vi "DCS(Dual_Inst).vi"(3 "error in":errorcluster) -> (10 "error out":errorcluster)   [LabVIEW 2013]
uses:
  <vilib>/Utility/miscctls.llb/LVPointTypeDef.ctl
  <userlib>/Accelerator/User Interface/Controls/Role ID.ctl
panel:
  out "Changed front panel":bool
  in  "stop":bool
  in  "Tab Control":enum32{"Engineering Graphs", "Maintenance"}(tab)
  out "DCS 2 Second Plane":ext[][](graph)
  out "DCS 2 First Plane":ext[][](graph)
  out "DCS 1 Second Plane":ext[][](graph)
  out "DCS 1 First Plane":ext[][](graph)
  out "DCS 1 Signals":ext[][](graph)
  out "DCS 2 Signals":ext[][](graph)
  out "Aquisition Rate Value 2":i64
  out "Aquisition Rate Value 1":i64
  out "DAQ 1 Sample Size Window":u32
  in  "DAQ 1 Trim Time":dbl=0.0001
  in  "DAQ 2 Trim Time":dbl=0.0001
  out "DAQ 2 Sample Size Window":i32
  in  "Save Waveforms":bool
  in  "Posttrigger size 2":i32=50000
  in  "Acquisition Rate 2":u16(ring)=2 items=["40 MHz", "20 MHz", "10 MHz", "5 MHz", "2.5 MHz", "1 MHz", "100 kHz", "10 kHz"]
  in  "Pretrigger size 2":i32=1
  in  "Rising or falling? 2":bool
  in  "Jorger 2 TR slot":i32=6
  out "Sampling Frequency":u16(ring) items=["40 MHz", "20 MHz", "10 MHz", "5 MHz", "2.5 MHz", "1 MHz", "100 kHz", "10 kHz"]
  out "Length of Sample":dbl caption="s" format="%^#_3g"
  out "Memory Address Pointer":ext
  out "Post trigger Size":ext
  out "Pretrigger Size":ext
  out "Trigger Generation register":i32=23 format="%.0b"
  out "status register":i8=4 format="%08b"
  out "control register":i16=23 format="%015b"
  in  "Posttrigger size":i32=1
  in  "Acquisition Rate":u16(ring)=2 items=["40 MHz", "20 MHz", "10 MHz", "5 MHz", "2.5 MHz", "1 MHz", "100 kHz", "10 kHz"]
  in  "Pretrigger size":i32=60000
  in  "Rising or falling?":bool
  out "Running Errors":errorcluster
  in  "Jorger 1 TR slot":i32=3
  in  "Joerger 1 Channels":i32[](array[numeric])=[0, 1, 2, 3, 4, 5, 6, 9]
  in  "Joerger 2 Channels":i32[](array[numeric])=[0, 1, 2, 3, 4, 6, 7, 8]
  out "control register 2":i16=23 format="%015b"
  out "status register 2":i8=4 format="%08b"
  out "Memory Address Pointer 2":ext
  out "Post trigger Size 2":ext
  out "Pretrigger Size 2":ext
  out "Sampling Frequency 2":u16(ring) items=["40 MHz", "20 MHz", "10 MHz", "5 MHz", "2.5 MHz", "1 MHz", "100 kHz", "10 kHz"]
  # "Ensure Joeger Card Channels are functional.\nDefault values should reflect this."
  # "Rising or falling? not functional. Ignore"
  # "DAQ 2 Parameter Controls"
  # "Falling"
  # "Rising"
  # "DAQ Parameter Indicators"
  # "DAQ 1 Parameter Controls"
  # "Falling"
  # "Rising"
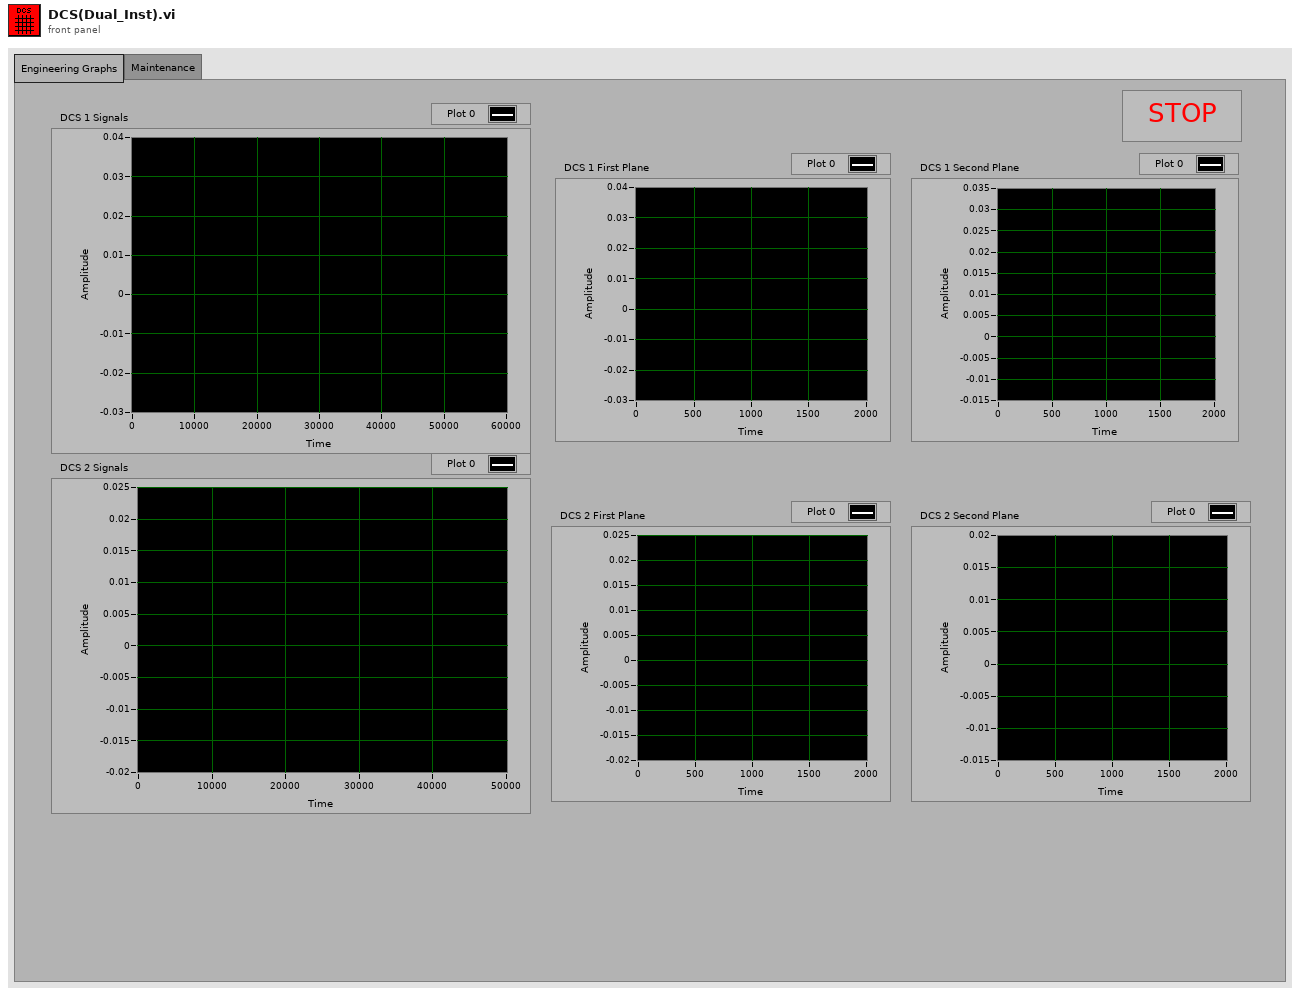
[diagram p1: front panel]
types:
  T1 = typedef "LVPointTypeDef.ctl" = cluster{"Horizontal":i16, "Vertical":i16}
  T2 = typedef "Role ID.ctl" = enum16{"First_Detector", "Second_Detector", "Third_Detector", "LeCroy_CH1", "LeCroy_CH2", "LeCroy_CH3", "LeCroy_CH4", "PSU", "DCS 1", "DCS 2"}
  T3 = enum32{"DCS", "Spot Size Tracking", "Engineering Graphs", "Maintenance"}
  T4 = cluster{"Data":dbl[][], "Integer Timestamp":u64, "Signal Length":u32, "DCS ID":u64, "Role ID":T2}
  T5 = cluster{"Data":dbl[][], "Integer Timestamp":u64, "Signal Length":u32, "DCS ID":u64, "Role ID":T2}[]
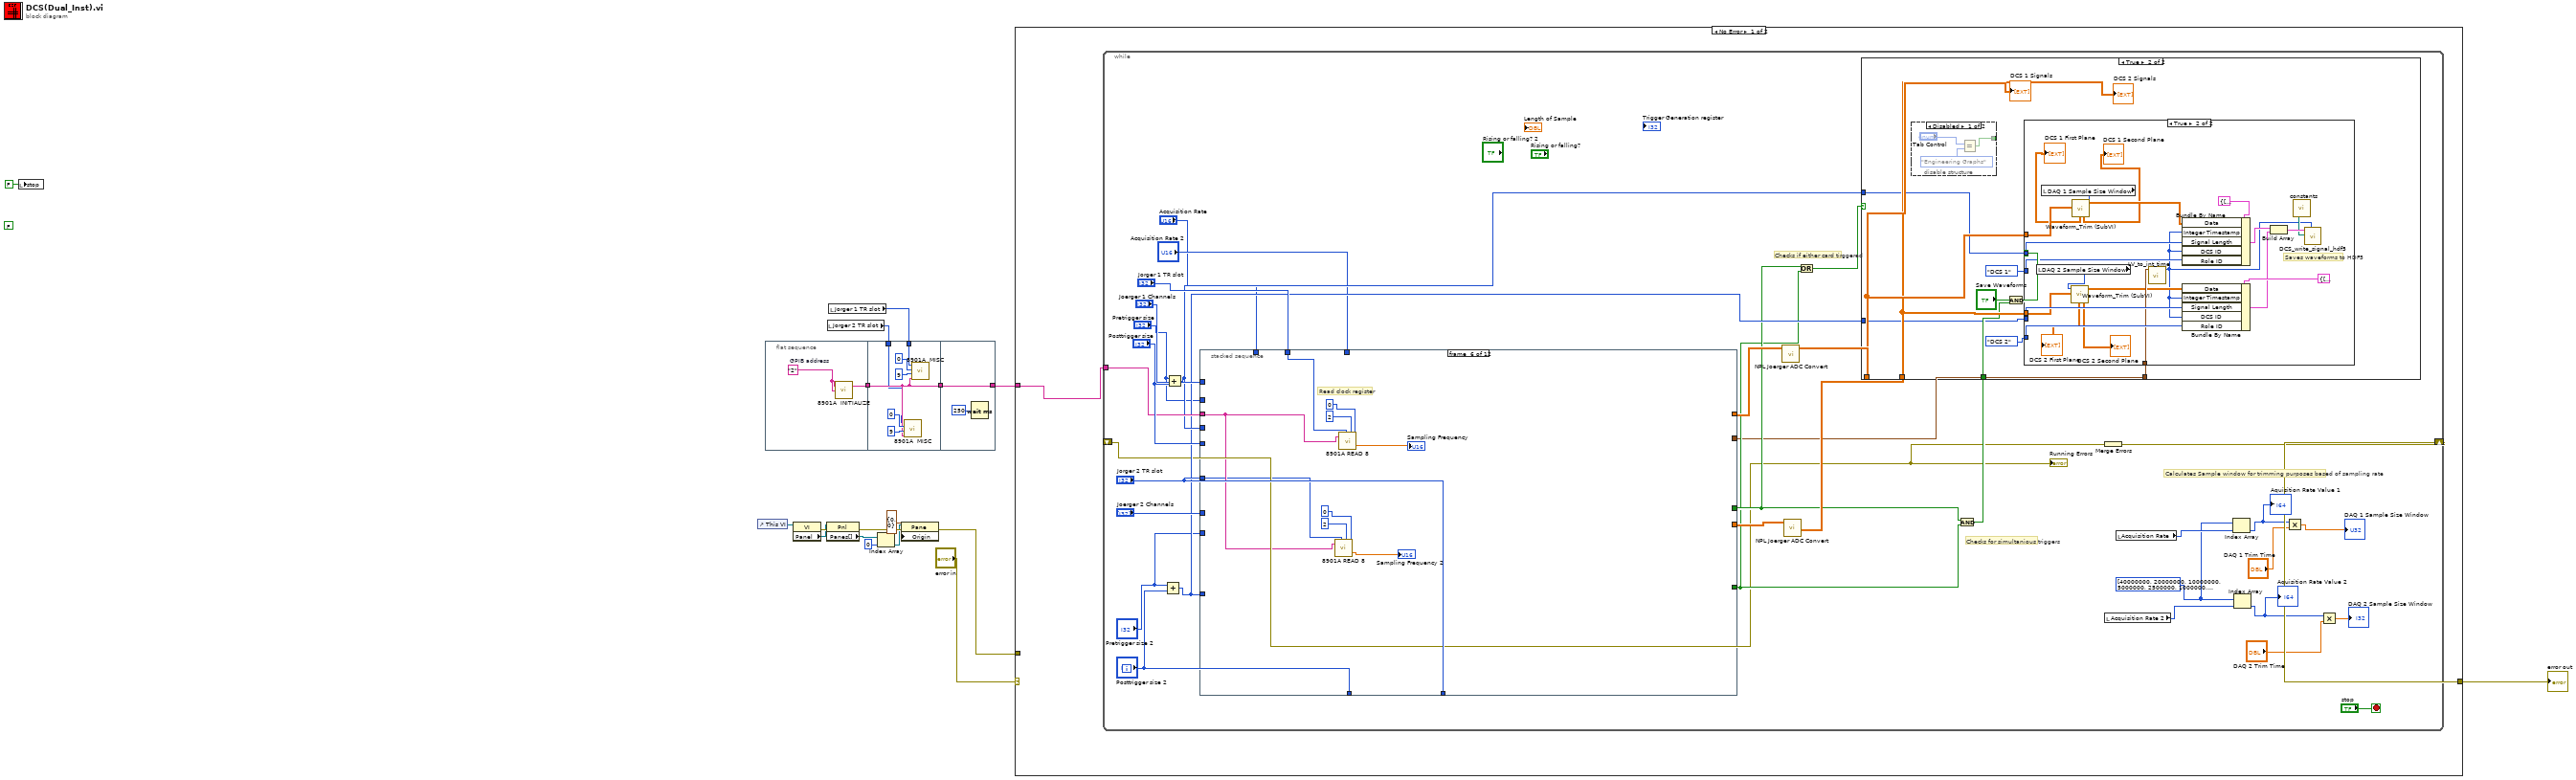
[diagram p0: block diagram]
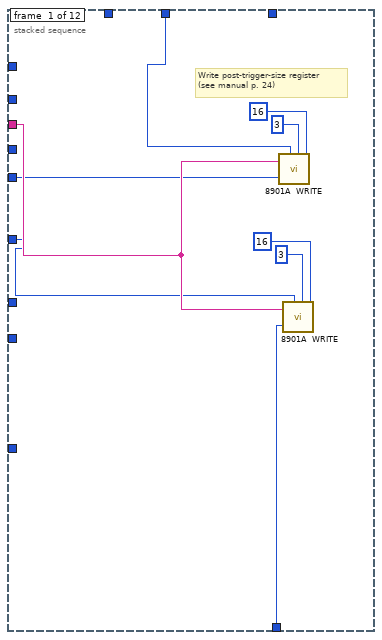
[diagram p5: hidden frame]
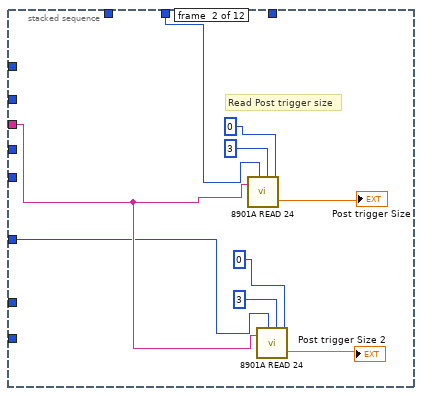
[diagram p6: hidden frame]
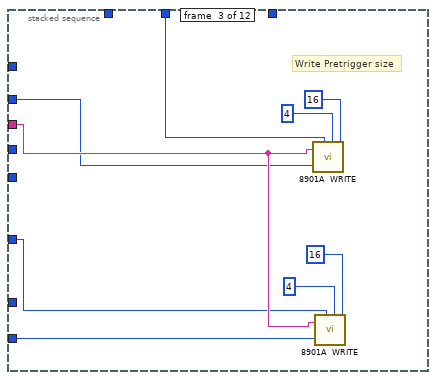
[diagram p7: hidden frame]
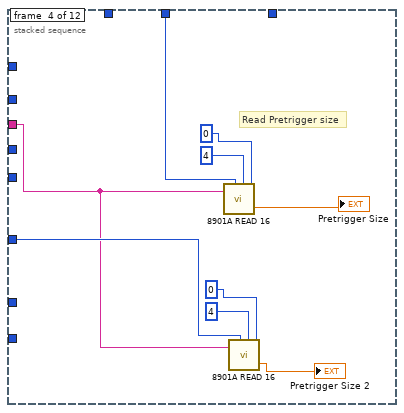
[diagram p8: hidden frame]
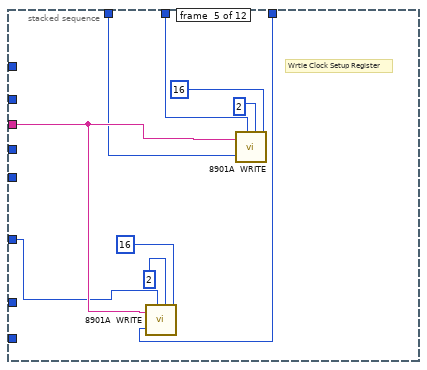
[diagram p9: hidden frame]
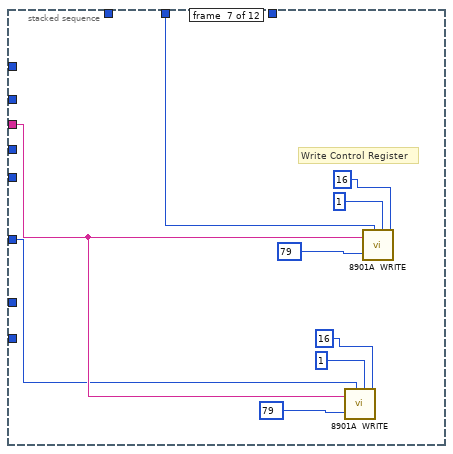
[diagram p10: hidden frame]
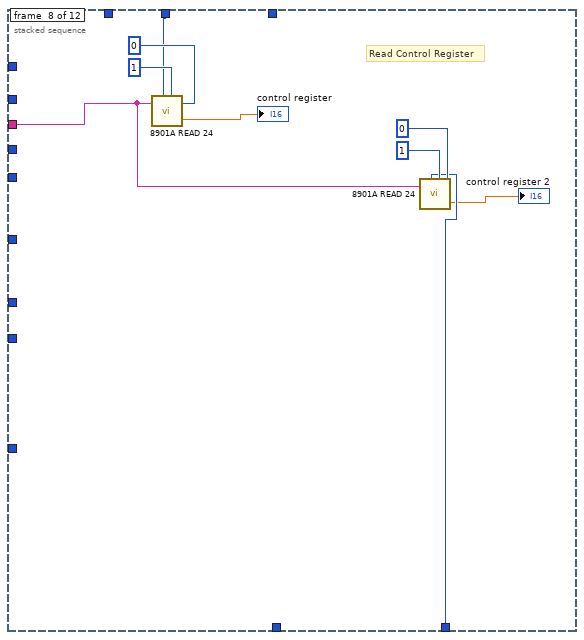
[diagram p11: hidden frame]
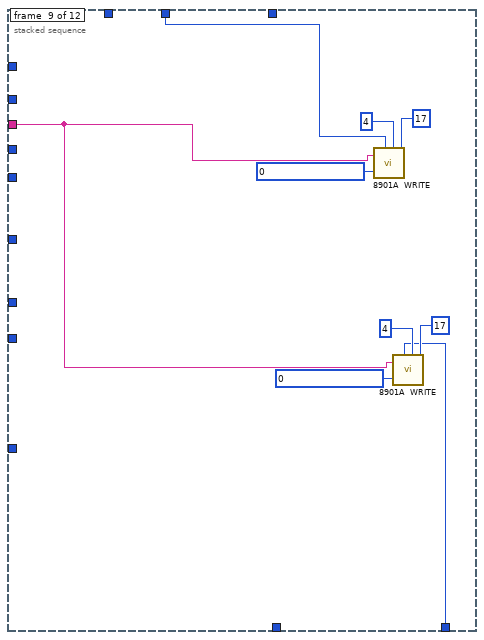
[diagram p12: hidden frame]
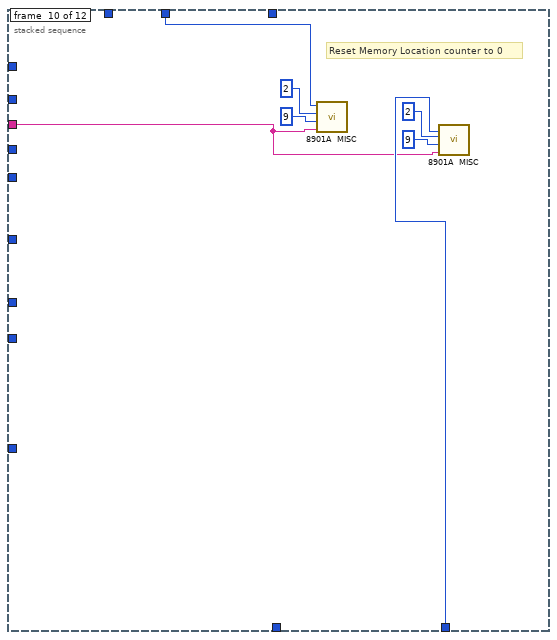
[diagram p13: hidden frame]
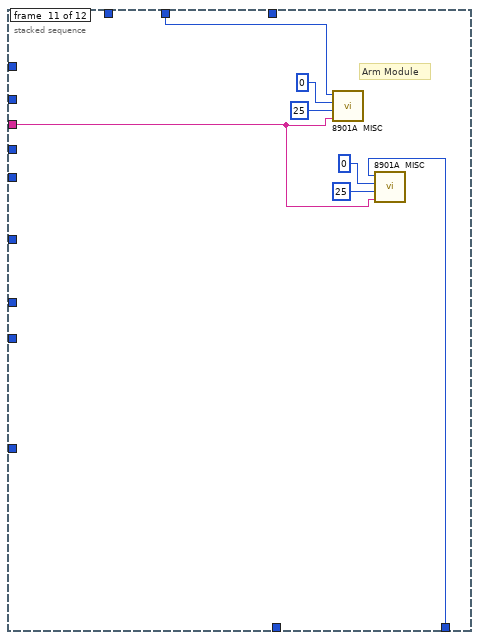
[diagram p14: hidden frame]
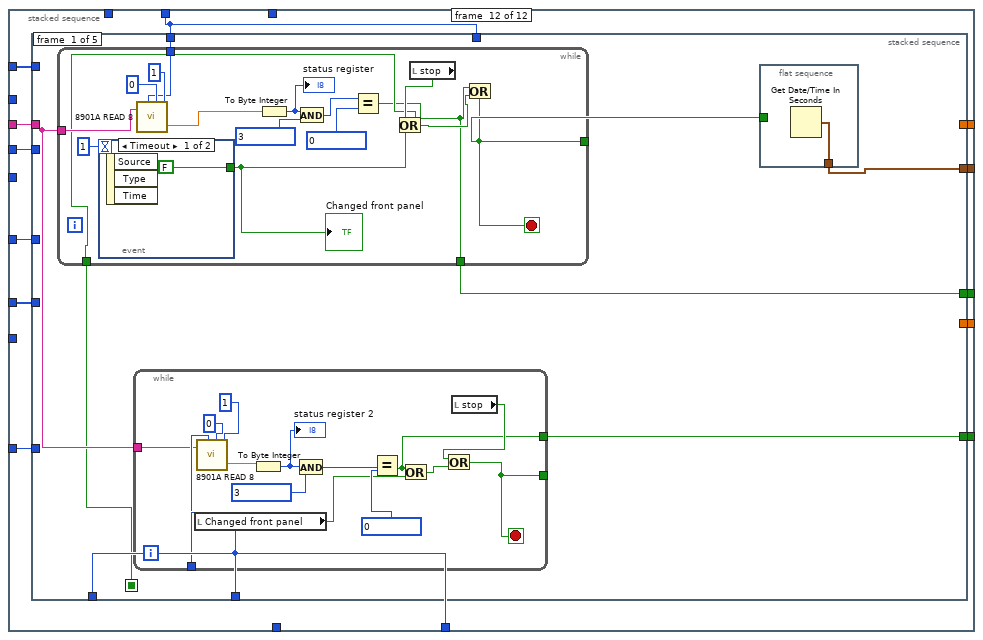
[diagram p15: hidden frame]
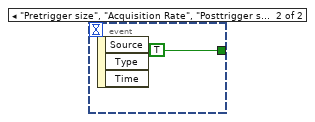
[diagram p16: hidden frame]
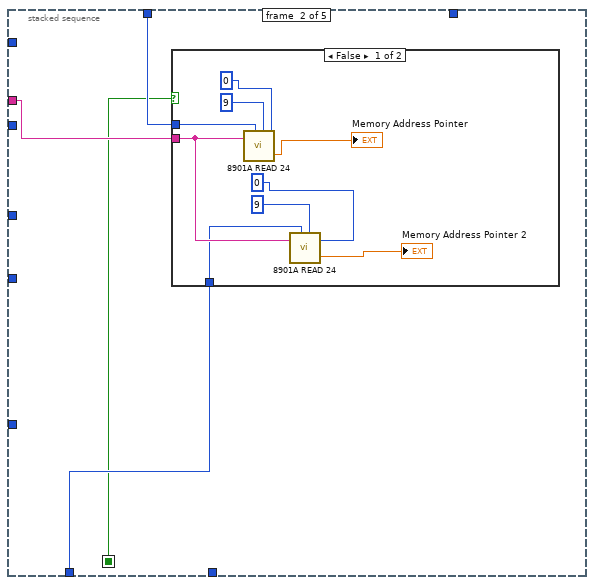
[diagram p17: hidden frame]
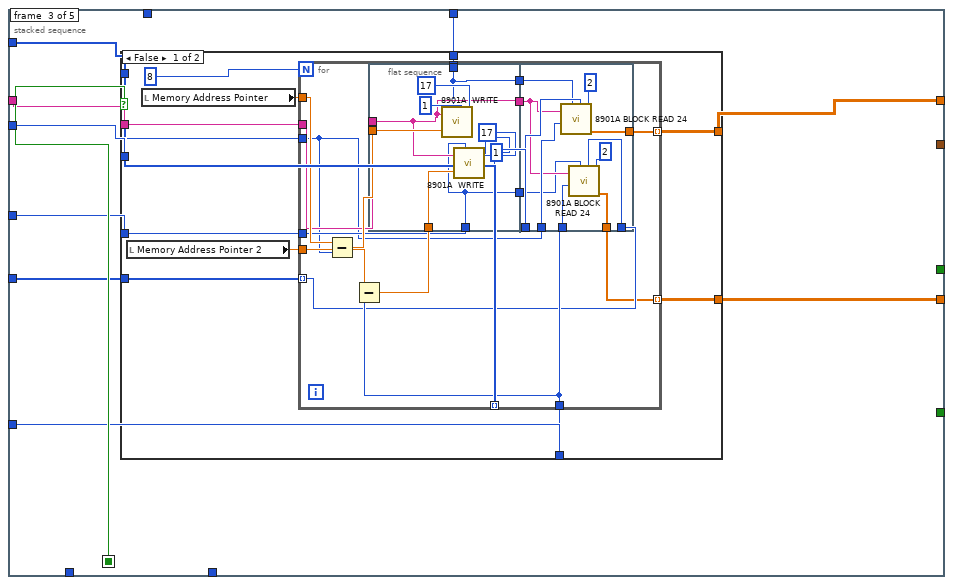
[diagram p19: hidden frame]
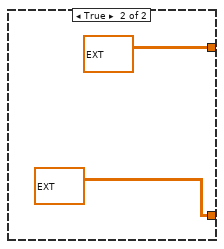
[diagram p20: hidden frame]
diagram:
  (unwired) FALSE ("Auto Threshold")
  n1 = local write "stop"(FALSE ("stop")) -> ()
  n2 = control-ref of="This VI"() -> (w14:refnum<vi>)
  n3 = flat-sequence {
    tunnel: [w18] -> w4
    tunnel: w4 -> [w21]
    tunnel: w3 -> [w20]
    tunnel: w2 -> [w19]
    tunnel: [w21] -> w1
    tunnel: [w27] -> w5
    tunnel: w1 -> [w27]
    frame #0 {
      w18 = "2"  # GPIB address
      n4 = call <instrlib>:"8901A  INITIALIZE.vi"("GPIB address"=w18) -> ()
    }
    frame #1 {
      n5 = call <instrlib>:"8901A  MISC.vi"("GPIB address"=w21, "f"=9, "a"=0, "n"=w19) -> ()
      n6 = call <instrlib>:"8901A  MISC.vi"("GPIB address"=w21, "f"=9, "a"=0, "n"=w20) -> ()
    }
    frame #2 {
      n7 = Wait (ms)(milliseconds to wait=250) -> ()  [unwired: 1 out]
    }
  }
  n8 = property class="VI"(reference=w14) -> (error out=w13:errorcluster, "Panel"=w12:refnum<vi>)  [unwired: 1 in, 1 out]
  n9 = property class="Pnl"(reference=w12, error in=w13) -> (error out=w11:errorcluster, "Panes[]"=w10:refnum<vi>[])  [unwired: 1 out]
  n10 = local read "Jorger 2 TR slot"() -> (w2:i32)
  n11 = local read "Jorger 1 TR slot"() -> (w3:i32)
  n12 = Index Array(array=w10, index=0) -> (element=w8:refnum<vi>)
  n13 = property class="Pane"(reference=w8, error in=w11, "Origin"=T1 {"Horizontal"=0, "Vertical"=0}) -> (error out=w6:errorcluster)  [unwired: 1 out]
  n14 = case shown="No Error" "error in" {
    selector: "error in" -> [_ w336]
    tunnel: [w29 w336] -> w16
    tunnel: w6 -> [_ _]
    tunnel: w5 -> [w28 _]
    frame No Error {
      n15 = while {
        shift-right: [w32] -> w29
        shift-left: _ -> [w33]
        tunnel: w28 -> [w53]
        stop <- "stop" stop-if-true
        w36 = i32[] [40000000, 20000000, 10000000, 5000000, 2500000, 1000000, 100000, 10000]
        # "Calculates Sample window for trimming purposes based of sampling rate"
        # "Checks if either card tirggered"
        # "Checks for simultanious triggers"
        n16 = Add(x="Pretrigger size 2", y="Posttrigger size 2") -> (x+y=w50:i32)
        n17 = Add(x="Pretrigger size", y="Posttrigger size") -> (x+y=w51:i32)
        n18 = stacked-sequence {
          tunnel: w53 -> [w103 w114 w121 w126 w139 w150 w154 w165 w173 w185 w189 w203]
          tunnel: w51 -> [_ _ _ _ _ _ _ _ _ _ _ w206]
          tunnel: "Joerger 1 Channels" -> [_ _ _ _ _ _ _ _ _ _ _ w205]
          tunnel: [_ _ _ _ _ _ _ _ _ _ _ w204] -> w61
          tunnel: "Jorger 2 TR slot" -> [_ _ _ _ _ _ _ w164 w171 w186 w188 w202]
          tunnel: "Jorger 1 TR slot" -> [w102 w110 w120 w130 w138 w148 w158 w162 w172 w184 w187 w195]
          tunnel: "Jorger 2 TR slot" -> [w101 w111 w119 w129 w137 w147 w153 _ _ _ _ w200]
          tunnel: "Posttrigger size" -> [w100 _ _ _ _ _ _ _ _ _ _ _]
          tunnel: "Posttrigger size 2" -> [w99 _ _ _ _ _ _ _ _ _ _ _]
          tunnel: "Acquisition Rate" -> [_ _ _ _ w136 _ _ _ _ _ _ _]
          tunnel: "Acquisition Rate 2" -> [_ _ _ _ w135 _ _ _ _ _ _ _]
          tunnel: w50 -> [_ _ _ _ _ _ _ _ _ _ _ w201]
          tunnel: "Joerger 2 Channels" -> [_ _ _ _ _ _ _ _ _ _ _ w199]
          tunnel: [_ _ _ _ _ _ _ _ _ _ _ w198] -> w52
          tunnel: [_ _ _ _ _ _ _ _ _ _ _ w197] -> w48
          tunnel: [_ _ _ _ _ _ _ _ _ _ _ w196] -> w47
          tunnel: "Pretrigger size 2" -> [_ _ w118 _ _ _ _ _ _ _ _ _]
          tunnel: "Pretrigger size" -> [_ _ w117 _ _ _ _ _ _ _ _ _]
          tunnel: [_ _ _ _ _ _ _ _ _ _ _ w194] -> w41
          frame #0 {
            # "Write post-trigger-size register\n(see manual p. 24)"
            n19 = call <instrlib>:"8901A  WRITE.vi"("data"=w100, "GPIB address"=w103, "n"=w102, "a"=3, "f"=16) -> ()  [unwired: 1 in]
            n20 = call <instrlib>:"8901A  WRITE.vi"("data"=w99, "GPIB address"=w103, "n"=w101, "a"=3, "f"=16) -> ()  [unwired: 1 in]
          }
          frame #1 {
            # "Read Post trigger size"
            n21 = call <instrlib>:"8901A READ 24.vi"("GPIB address"=w114, "n"=w110, "a"=3, "f"=0) -> ("output"=→"Post trigger Size":ext)  [unwired: 3 in]
            n22 = call <instrlib>:"8901A READ 24.vi"("GPIB address"=w114, "n"=w111, "a"=3, "f"=0) -> ("output"=→"Post trigger Size 2":ext)  [unwired: 3 in]
          }
          frame #2 {
            # "Write Pretrigger size"
            n23 = call <instrlib>:"8901A  WRITE.vi"("data"=w117, "GPIB address"=w121, "n"=w120, "a"=4, "f"=16) -> ()  [unwired: 1 in]
            n24 = call <instrlib>:"8901A  WRITE.vi"("data"=w118, "GPIB address"=w121, "n"=w119, "a"=4, "f"=16) -> ()  [unwired: 1 in]
          }
          frame #3 {
            # "Read Pretrigger size"
            n25 = call <instrlib>:"8901A READ 16.vi"("GPIB address"=w126, "n"=w130, "a"=u8 4, "f"=u8 0) -> ("output"=→"Pretrigger Size":ext)  [unwired: 3 in]
            n26 = call <instrlib>:"8901A READ 16.vi"("GPIB address"=w126, "n"=w129, "a"=u8 4, "f"=u8 0) -> ("output"=→"Pretrigger Size 2":ext)  [unwired: 3 in]
          }
          frame #4 {
            # "Wrtie Clock Setup Register"
            n27 = call <instrlib>:"8901A  WRITE.vi"("data"=w135, "GPIB address"=w139, "n"=w137, "a"=2, "f"=16) -> ()  [unwired: 1 in]
            n28 = call <instrlib>:"8901A  WRITE.vi"("data"=w136, "GPIB address"=w139, "n"=w138, "a"=2, "f"=16) -> ()  [unwired: 1 in]
          }
          frame #5 {
            # "Read clock register"
            n29 = call <instrlib>:"8901A READ 8.vi"("GPIB address"=w150, "n"=w147, "a"=2, "f"=0) -> ("output"=→"Sampling Frequency 2":ext)  [unwired: 3 in]
            n30 = call <instrlib>:"8901A READ 8.vi"("GPIB address"=w150, "n"=w148, "a"=2, "f"=0) -> ("output"=→"Sampling Frequency":ext)  [unwired: 3 in]
          }
          frame #6 {
            # "Write Control Register"
            n31 = call <instrlib>:"8901A  WRITE.vi"("data"=79, "GPIB address"=w154, "n"=w153, "a"=1, "f"=16) -> ()  [unwired: 1 in]
            n32 = call <instrlib>:"8901A  WRITE.vi"("data"=79, "GPIB address"=w154, "n"=w158, "a"=1, "f"=16) -> ()  [unwired: 1 in]
          }
          frame #7 {
            # "Read Control Register"
            n33 = call <instrlib>:"8901A READ 24.vi"("GPIB address"=w165, "n"=w162, "a"=1, "f"=0) -> ("output"=→"control register":ext)  [unwired: 3 in]
            n34 = call <instrlib>:"8901A READ 24.vi"("GPIB address"=w165, "n"=w164, "a"=1, "f"=0) -> ("output"=→"control register 2":ext)  [unwired: 3 in]
          }
          frame #8 {
            n35 = call <instrlib>:"8901A  WRITE.vi"("data"=0, "GPIB address"=w173, "n"=w172, "a"=u8 4, "f"=u8 17) -> ()  [unwired: 1 in]
            n36 = call <instrlib>:"8901A  WRITE.vi"("data"=0, "GPIB address"=w173, "n"=w171, "a"=u8 4, "f"=u8 17) -> ()  [unwired: 1 in]
          }
          frame #9 {
            # "Reset Memory Location counter to 0"
            n37 = call <instrlib>:"8901A  MISC.vi"("GPIB address"=w185, "f"=u8 9, "a"=u8 2, "n"=w184) -> ()
            n38 = call <instrlib>:"8901A  MISC.vi"("GPIB address"=w185, "f"=u8 9, "a"=u8 2, "n"=w186) -> ()
          }
          frame #10 {
            # "Arm Module"
            n39 = call <instrlib>:"8901A  MISC.vi"("GPIB address"=w189, "f"=25, "a"=0, "n"=w187) -> ()
            n40 = call <instrlib>:"8901A  MISC.vi"("GPIB address"=w189, "f"=25, "a"=0, "n"=w188) -> ()
          }
          frame #11 {
            n41 = stacked-sequence {
              seq-local: [w212 _ _ _ _] -> [_ w247 w269 _ _]
              tunnel: w206 -> [_ _ w268 _ _]
              tunnel: w205 -> [_ _ w267 _ _]
              tunnel: [_ _ w265 _ _] -> w204
              tunnel: w202 -> [w214 _ _ w321 _]
              tunnel: w203 -> [w213 w250 w266 w322 w331]
              tunnel: w202 -> [_ w249 _ _ _]
              tunnel: w201 -> [_ _ w264 _ _]
              tunnel: w195 -> [_ _ w263 _ w330]
              tunnel: w200 -> [_ _ w261 _ w329]
              tunnel: w199 -> [_ _ w262 _ _]
              tunnel: [_ _ w260 _ _] -> w198
              tunnel: [w211 _ _ _ _] -> w197
              tunnel: [w210 _ _ _ _] -> w196
              tunnel: w195 -> [w209 w248 _ w325 _]
              tunnel: [w207 _ _ _ _] -> w194
              frame #0 {
                n42 = while {
                  tunnel: w213 -> [w237]
                  tunnel: [w235] -> w208
                  tunnel: [w231] -> w212
                  tunnel: [w230] -> w211
                  tunnel: w209 -> [w229]
                  stop <- w235 stop-if-true
                  n43 = event shown="[0] Timeout" {
                    selector: _ -> [_ _]
                    dyn-events: _ -> [_ _]
                    timeout: 1 -> [_ _]
                    tunnel: [FALSE TRUE] -> w233
                    event Timeout {
                      n44 = event-data() -> ()  [unwired: 1 in, 3 out]
                    }
                    event "Pretrigger size", "Acquisition Rate", "Posttrigger size", "control register": Value Change {
                      n45 = event-data() -> ()  [unwired: 1 in, 3 out]
                    }
                  }
                  "Changed front panel" <- w233
                  n46 = call <instrlib>:"8901A READ 8.vi"("GPIB address"=w237, "n"=w229, "a"=0, "f"=1) -> ("output"=w240:ext)  [unwired: 3 in]
                  n47 = To Byte Integer(number=w240) -> (8bit integer=w236:i8)
                  "status register" <- w236
                  n48 = And(x=w236, y=i8 3) -> (x .and. y?=w241:i8)
                  n49 = Equal?(x=w241, y=i8 0) -> (x = y?=w230:bool)
                  n50 = local read "stop"() -> (w232:bool)
                  n51 = Or(x=w232, y=w233) -> (x .or. y?=w231:bool)
                  n52 = Or(x=w230, y=w231) -> (x .or. y?=w235:bool)
                }
                n53 = while {
                  tunnel: w214 -> [w226]
                  tunnel: w213 -> [w225]
                  tunnel: [w218] -> _
                  tunnel: [w215] -> w210
                  stop <- w218 stop-if-true
                  n54 = local read "Changed front panel"() -> (w216:bool)
                  n55 = call <instrlib>:"8901A READ 8.vi"("GPIB address"=w225, "n"=w226, "a"=0, "f"=1) -> ("output"=w224:ext)  [unwired: 3 in]
                  n56 = To Byte Integer(number=w224) -> (8bit integer=w220:i8)
                  "status register 2" <- w220
                  n57 = And(x=w220, y=i8 3) -> (x .and. y?=w222:i8)
                  n58 = Equal?(x=w222, y=i8 0) -> (x = y?=w215:bool)
                  n59 = Or(x=w215, y=w216) -> (x .or. y?=w217:bool)
                  n60 = local read "stop"() -> (w219:bool)
                  n61 = Or(x=w219, y=w217) -> (x .or. y?=w218:bool)
                }
                n62 = flat-sequence {
                  tunnel: w208 -> [_]
                  tunnel: [w246] -> w207
                  frame #0 {
                    n63 = Get Date/Time In Seconds() -> (seconds since 1Jan1904=w246:timestamp)
                  }
                }
              }
              frame #1 {
                n64 = case shown="False" w247 {
                  tunnel: w250 -> [w254 _]
                  tunnel: w249 -> [w253 _]
                  tunnel: w248 -> [w251 _]
                  frame False {
                    n65 = call <instrlib>:"8901A READ 24.vi"("GPIB address"=w254, "n"=w251, "a"=u8 9, "f"=u8 0) -> ("output"=→"Memory Address Pointer":ext)  [unwired: 3 in]
                    n66 = call <instrlib>:"8901A READ 24.vi"("GPIB address"=w254, "n"=w253, "a"=u8 9, "f"=u8 0) -> ("output"=→"Memory Address Pointer 2":ext)  [unwired: 3 in]
                  }
                  frame True {
                  }
                }
              }
              frame #2 {
                n67 = case shown="False" w269 {
                  tunnel: w268 -> [w279 _]
                  tunnel: w267 -> [w280 _]
                  tunnel: w266 -> [w278 _]
                  tunnel: [w276 ext[][] [[nan]] ("output")] -> w265
                  tunnel: w264 -> [w275 _]
                  tunnel: w263 -> [w273 _]
                  tunnel: w261 -> [w272 _]
                  tunnel: w262 -> [w271 _]
                  tunnel: [w270 ext[][] [[nan]] ("output")] -> w260
                  frame False {
                    n68 = local read "Memory Address Pointer 2"() -> (w274:ext)
                    n69 = local read "Memory Address Pointer"() -> (w277:ext)
                    n70 = for {
                      N: 8 -> [_]
                      tunnel: w280 -> [w293] mode=indexing
                      tunnel: w279 -> [w284]
                      tunnel: w278 -> [w295]
                      tunnel: w277 -> [w297]
                      tunnel: [w292] -> w276 mode=indexing
                      tunnel: w275 -> [w290]
                      tunnel: w274 -> [w291]
                      tunnel: w273 -> [w288]
                      tunnel: w272 -> [w287]
                      tunnel: w271 -> [w283] mode=indexing
                      tunnel: [w282] -> w270 mode=indexing
                      n71 = Subtract(x=w297, y=w284) -> (x-y=w296:ext)
                      n72 = Subtract(x=w291, y=w290) -> (x-y=w289:ext)
                      n73 = flat-sequence {
                        tunnel: w296 -> [w304]
                        tunnel: w295 -> [w302]
                        tunnel: [w302] -> w294
                        tunnel: w289 -> [w303]
                        tunnel: w288 -> [w298]
                        tunnel: w287 -> [w299]
                        tunnel: [w298] -> w286
                        tunnel: [w299] -> w285
                        tunnel: w294 -> [w310]
                        tunnel: w293 -> [w312]
                        tunnel: w284 -> [w316]
                        tunnel: [w315] -> w292
                        tunnel: w290 -> [w313]
                        tunnel: w286 -> [w307]
                        tunnel: w285 -> [w308]
                        tunnel: w283 -> [w311]
                        tunnel: [w309] -> w282
                        frame #0 {
                          n74 = call <instrlib>:"8901A  WRITE.vi"("data"=w304, "GPIB address"=w302, "n"=w298, "a"=1, "f"=17) -> ()  [unwired: 1 in]
                          n75 = call <instrlib>:"8901A  WRITE.vi"("data"=w303, "GPIB address"=w302, "n"=w299, "a"=1, "f"=17) -> ()  [unwired: 1 in]
                        }
                        frame #1 {
                          n76 = call <instrlib>:"8901A BLOCK READ 24.vi"("f"=2, "a"=w312, "n"=w307, "GPIB address"=w310, "# points to read"=w316) -> ("output"=w315:ext[])  [unwired: 4 in]
                          n77 = call <instrlib>:"8901A BLOCK READ 24.vi"("f"=2, "a"=w311, "n"=w308, "GPIB address"=w310, "# points to read"=w313) -> ("output"=w309:ext[])  [unwired: 4 in]
                        }
                      }
                    }
                  }
                  frame True {
                  }
                }
              }
              frame #3 {
                # "Read in control register"
                n78 = call <instrlib>:"8901A READ 24.vi"("GPIB address"=w322, "n"=w325, "a"=1, "f"=0) -> ("output"=w326:ext)  [unwired: 3 in]
                n79 = call <instrlib>:"8901A READ 24.vi"("GPIB address"=w322, "n"=w321, "a"=1, "f"=0) -> ("output"=w320:ext)  [unwired: 3 in]
                n80 = local write "control register"(w326) -> ()
                n81 = local write "control register 2"(w320) -> ()
              }
              frame #4 {
                # "Abort Readout"
                n82 = call <instrlib>:"8901A  MISC.vi"("GPIB address"=w331, "f"=25, "a"=2, "n"=w329) -> ()
                n83 = call <instrlib>:"8901A  MISC.vi"("GPIB address"=w331, "f"=25, "a"=2, "n"=w330) -> ()
              }
            }
          }
        }
        n84 = call <userlib>:"NPL Joerger ADC Convert.vi"("Input"=w61) -> ("Output"=w60:ext[][])  [unwired: 10 in]
        n85 = call <userlib>:"NPL Joerger ADC Convert.vi"("Input"=w52) -> ("Output"=w59:ext[][])  [unwired: 10 in]
        n86 = Or(x=w48, y=w47) -> (x .or. y?=w46:bool)
        n87 = And(x=w48, y=w47) -> (x .and. y?=w49:bool)
        n88 = case shown="True" w46 {
          tunnel: w60 -> [_ w72]
          tunnel: w51 -> [_ w70]
          tunnel: w59 -> [_ w71]
          tunnel: w49 -> [_ w66]
          tunnel: w50 -> [_ w65]
          tunnel: w41 -> [_ w64]
          frame False {
          }
          frame True {
            n89 = disable-structure shown="Disabled" {
              disable-tunnel: [w74 _] -> _
              frame Disabled {
                n90 = Equal?(x="Tab Control", y=T3."Engineering Graphs") -> (x = y?=w74:bool)
              }
              frame Enabled {
              }
            }
            n91 = And(x="Save Waveforms", y=w66) -> (x .and. y?=w67:bool)
            n92 = case shown="True" w67 {
              tunnel: Role_ID."DCS 1" ("Role ID") -> [_ w95]
              tunnel: w70 -> [_ w94]
              tunnel: w72 -> [_ w88]
              tunnel: w71 -> [_ w86]
              tunnel: w65 -> [_ w91]
              tunnel: Role_ID."DCS 2" ("Role ID") -> [_ w90]
              tunnel: w64 -> [_ w89]
              frame False {
              }
              frame True {
                # "Saves waveforms to HDF5"
                n93 = local read "DAQ 2 Sample Size Window"() -> (w83:i32)
                n94 = local read "DAQ 1 Sample Size Window"() -> (w84:u32)
                n95 = call <userlib>:"Waveform_Trim (SubVI).vi"("Raw Waveform"=w86, "DAQ Sample Window"=w83) -> ("Trimmed Waveform"=w85:ext[][], "Second Plane"=→"DCS 2 Second Plane":ext[][], "First Plane"=→"DCS 2 First Plane":ext[][])  [unwired: 5 in, 2 out]
                n96 = call <userlib>:"Waveform_Trim (SubVI).vi"("Raw Waveform"=w88, "DAQ Sample Window"=w84) -> ("Trimmed Waveform"=w87:ext[][], "Second Plane"=→"DCS 1 Second Plane":ext[][], "First Plane"=→"DCS 1 First Plane":ext[][])  [unwired: 5 in, 2 out]
                n97 = call <userlib>:"LV_to_int_time.vi"("Time Stamp"=w89) -> ("Integer Time"=w77:i64)  [unwired: 8 in, 1 out]
                n98 = Bundle By Name(cluster=T4 {"Data"=[], "Integer Timestamp"=0, "Signal Length"=0, "DCS ID"=0, "Role ID"=enum."First_Detector"} ("Cluster"), "Data"=w87, "Integer Timestamp"=w77, "Signal Length"=w94, "DCS ID"=w77, "Role ID"=w95) -> (w97:T4)
                n99 = Bundle By Name(cluster=T4 {"Data"=[], "Integer Timestamp"=0, "Signal Length"=0, "DCS ID"=0, "Role ID"=enum."First_Detector"} ("Cluster"), "Data"=w85, "Integer Timestamp"=w77, "Signal Length"=w91, "DCS ID"=w77, "Role ID"=w90) -> (w92:T4)
                n100 = Build Array(w97, w92) -> (w96:T5)
                n101 = call <userlib>:"constants.vi"() -> ("DCS Temp filepath"=w82:path)  [unwired: 3 out]
                n102 = call <userlib>:"DCS_write_signal_hdf5.vi"("Index"=w77, "Save Path"=w82, "Signal array"=w96) -> ()  [unwired: 8 in, 1 out]
              }
            }
            "DCS 1 Signals" <- w72
            "DCS 2 Signals" <- w71
          }
        }
        n103 = Merge Errors(w33) -> (w32:errorcluster)
        n104 = local read "Acquisition Rate 2"() -> (w38:u16)
        n105 = local read "Acquisition Rate"() -> (w37:u16)
        n106 = Index Array(array=w36, index=w37) -> (element=w30:i32)
        "Aquisition Rate Value 1" <- w30
        n107 = Index Array(array=w36, index=w38) -> (element=w31:i32)
        "Aquisition Rate Value 2" <- w31
        n108 = Multiply(x=w30, y="DAQ 1 Trim Time") -> (x*y=→"DAQ 1 Sample Size Window":dbl)
        n109 = Multiply(x=w31, y="DAQ 2 Trim Time") -> (x*y=→"DAQ 2 Sample Size Window":dbl)
        "Running Errors" <- w33
      }
    }
    frame Error {
    }
  }
  "error out" <- w16
